vi "GPSGSA.vi"(1 "String":string) -> (0 "Array":string[](array[string]))   [LabVIEW 2020]
panel:
  out "Satelite 9":string
  out "Satelite 10":string
  out "Satelite 11":string
  out "Satelite 12":string
  out "Satelite 7":string
  out "Satelite 8":string
  out "Satelite 6":string
  out "Satelite 5":string
  out "Satelite 4":string
  out "Satelite 3":string
  out "Satelite 2":string
  out "Satelite 1":string
  out "FIX STATUS":string
  out "MODO":string
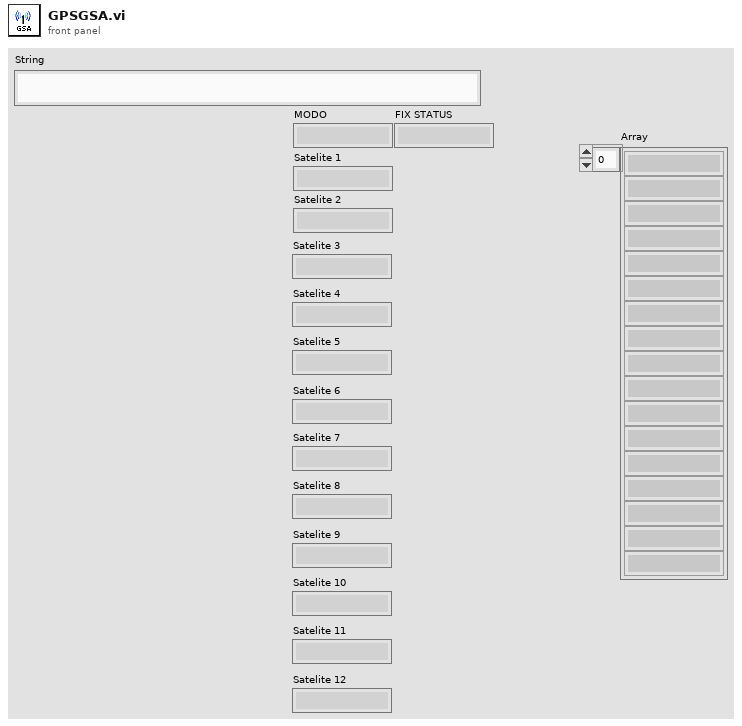
[diagram p1: front panel]
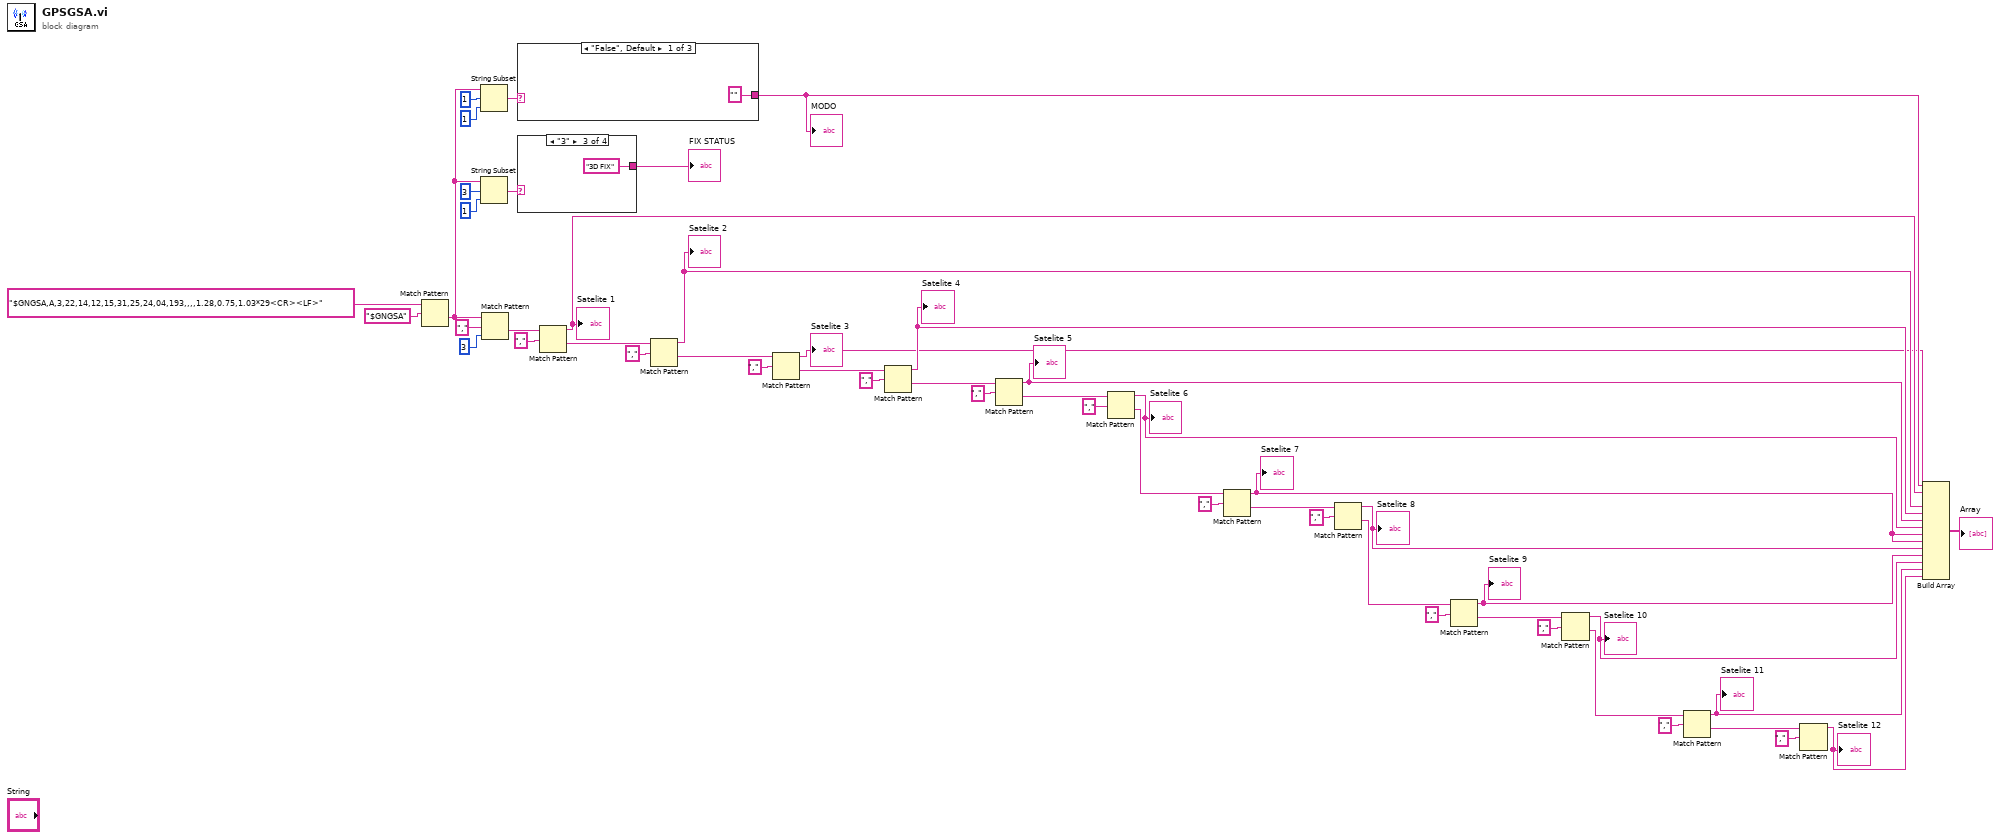
[diagram p0: block diagram]
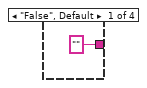
[diagram p2: hidden frame]
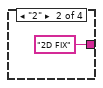
[diagram p3: hidden frame]
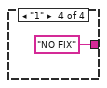
[diagram p4: hidden frame]
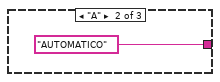
[diagram p5: hidden frame]
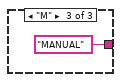
[diagram p6: hidden frame]
diagram:
  n1 = Match Pattern(string="$GNGSA,A,3,22,14,12,15,31,25,24,04,193,,,,1.28,0.75,1.03*29<CR><LF>", regular expression="$GNGSA") -> (after substring=w41:string)  [unwired: 1 in, 3 out]
  n2 = String Subset(string=w41, offset (0)=1, length (rest)=1 ("length (rest)")) -> (substring=w46:string)
  n3 = String Subset(string=w41, offset (0)=3, length (rest)=1 ("length (rest)")) -> (substring=w43:string)
  n4 = Match Pattern(string=w41, regular expression=",", offset (0)=3) -> (after substring=w38:string)  [unwired: 3 out]
  n5 = case shown="\"False\", Default" w46 {
    tunnel: ["" "AUTOMATICO" "MANUAL"] -> w3
    frame "False", Default {
    }
    frame "A" {
    }
    frame "M" {
    }
  }
  "MODO" <- w3
  n6 = case shown="\"3\"" w43 {
    tunnel: ["" "2D FIX" "3D FIX" "NO FIX"] -> w42
    frame "False", Default {
    }
    frame "2" {
    }
    frame "3" {
    }
    frame "1" {
    }
  }
  "FIX STATUS" <- w42
  n7 = Match Pattern(string=w38, regular expression=",") -> (before substring=w2:string, after substring=w36:string)  [unwired: 1 in, 2 out]
  "Satelite 1" <- w2
  n8 = Match Pattern(string=w36, regular expression=",") -> (before substring=w14:string, after substring=w34:string)  [unwired: 1 in, 2 out]
  "Satelite 2" <- w14
  n9 = Match Pattern(string=w34, regular expression=",") -> (before substring=w1:string, after substring=w31:string)  [unwired: 1 in, 2 out]
  "Satelite 3" <- w1
  n10 = Match Pattern(string=w31, regular expression=",") -> (before substring=w12:string, after substring=w29:string)  [unwired: 1 in, 2 out]
  "Satelite 4" <- w12
  n11 = Match Pattern(string=w29, regular expression=",") -> (before substring=w11:string, after substring=w27:string)  [unwired: 1 in, 2 out]
  "Satelite 5" <- w11
  n12 = Match Pattern(string=w27, regular expression=",") -> (before substring=w10:string, after substring=w23:string)  [unwired: 1 in, 2 out]
  "Satelite 6" <- w10
  n13 = Match Pattern(string=w23, regular expression=",") -> (before substring=w9:string, after substring=w26:string)  [unwired: 1 in, 2 out]
  "Satelite 7" <- w9
  n14 = Match Pattern(string=w26, regular expression=",") -> (before substring=w8:string, after substring=w16:string)  [unwired: 1 in, 2 out]
  "Satelite 8" <- w8
  n15 = Match Pattern(string=w16, regular expression=",") -> (before substring=w7:string, after substring=w18:string)  [unwired: 1 in, 2 out]
  "Satelite 9" <- w7
  n16 = Match Pattern(string=w18, regular expression=",") -> (before substring=w6:string, after substring=w22:string)  [unwired: 1 in, 2 out]
  "Satelite 10" <- w6
  n17 = Match Pattern(string=w22, regular expression=",") -> (before substring=w5:string, after substring=w19:string)  [unwired: 1 in, 2 out]
  "Satelite 11" <- w5
  n18 = Match Pattern(string=w19, regular expression=",") -> (before substring=w4:string)  [unwired: 1 in, 3 out]
  "Satelite 12" <- w4
  n19 = Build Array(w3, w2, w1, w14, w12, w11, w10, w9, w9, w8, w7, w6, w5, w4) -> (→"Array":string[])
